vi "Eval X-Y-Z(a,t1,t2).vi"(5 "Variables":string[](array[string])=["t1", "t2"], 6 "Formulas":string[](array[string])=["", "", ""], 7 "Parameters":cluster{"name":string, "value":dbl}[](array[cluster]) {"value" format="%.2f"}, 8 "number of points":u32=25, 9 "End":dbl[](array[numeric])=[1.0, 1.0] format="%.2f", 10 "Start":dbl[](array[numeric])=[0.0, 0.0] format="%.2f") -> (0 "error":i32, 1 "ticks":u32, 2 "Z":dbl[](array[numeric]) format="%.2f", 3 "Y":dbl[](array[numeric]) format="%.2f", 4 "X":dbl[](array[numeric]) format="%.2f")   [LabVIEW 2020, in "NI_Gmath.lvlib"]
doc: "Describes a surface in 3D with two variables running over two different intervals."
uses:
  NI_Gmath.lvlib
panel:
  # "Example:\n\n number of points: 25 \n Start: 0.0 and 0.0\n End: 1.0 and 1.0\n Parameters: (a,1) and (b,2) \n Variables: t1 and t2\n Formulas: a*sin(t1) and a*cos(t1+t2) and b+exp(-t2)"
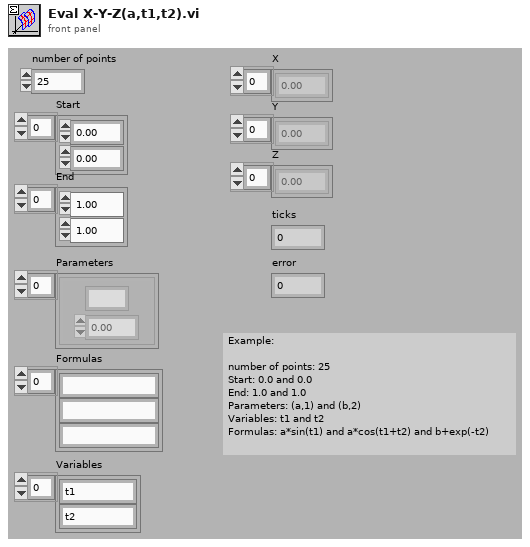
[diagram p1: front panel]
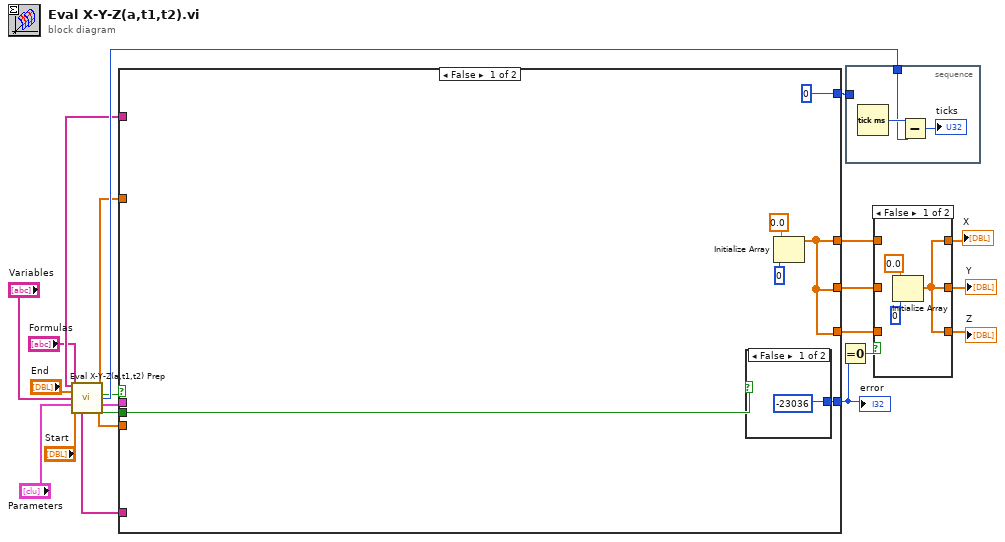
[diagram p0: block diagram]
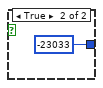
[diagram p3: hidden frame]
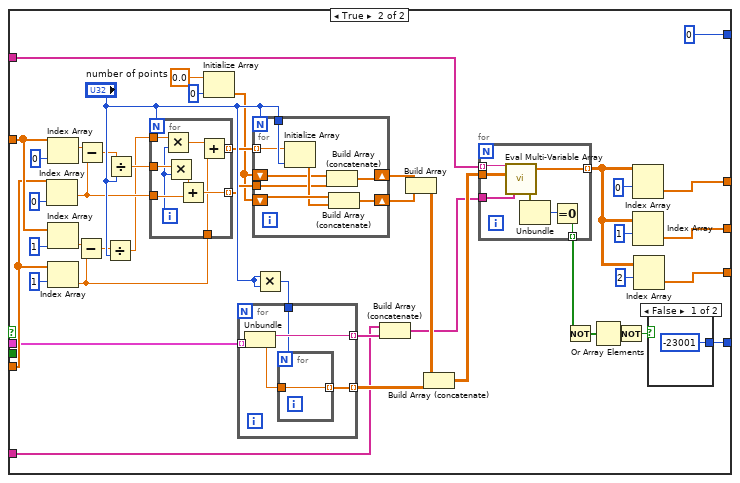
[diagram p4: hidden frame]
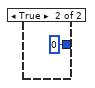
[diagram p5: hidden frame]
diagram:
  n1 = call "Eval X-Y-Z(a,t1,t2) Prep.vi"("End"="End", "Formulas"="Formulas", "Variables"="Variables", "Parameters"="Parameters", "Start"="Start") -> ("Formulas"=w17:string[], "End"=w19:dbl[], "time [msec]"=w21:u32, "error (general)"=w20:bool, "Variables"=w6:string[], "Start"=w18:dbl[], "Parameters"=w8:cluster{string, dbl}[], "specific error situation"=w7:bool)  [unwired: 3 in]
  n2 = case shown="False" w20 {
    tunnel: [0 0] -> w22
    tunnel: [w25 w43] -> w14
    tunnel: [w25 w42] -> w12
    tunnel: w19 -> [_ w41]
    tunnel: w18 -> [_ w40]
    tunnel: w6 -> [_ w39]
    tunnel: w8 -> [_ w38]
    tunnel: w17 -> [_ w37]
    tunnel: [w24 w34] -> w16
    tunnel: [w25 w33] -> w10
    tunnel: w7 -> [w23 _]
    frame False {
      n3 = case shown="False" w23 {
        tunnel: [-23036 -23033] -> w24
        frame False {
        }
        frame True {
        }
      }
      n4 = Initialize Array(0.0, 0) -> (w25:dbl[])
    }
    frame True {
      n5 = Index Array(array=w40, index=0) -> (element=w60:dbl)
      n6 = Index Array(array=w41, index=0) -> (element=w59:dbl)
      n7 = Index Array(array=w41, index=1) -> (element=w61:dbl)
      n8 = Index Array(array=w40, index=1) -> (element=w62:dbl)
      n9 = Subtract(x=w61, y=w62) -> (x-y=w51:dbl)
      n10 = Subtract(x=w59, y=w60) -> (x-y=w44:dbl)
      n11 = Divide(x=w51, y="number of points") -> (x/y=w53:dbl)
      n12 = Divide(x=w44, y="number of points") -> (x/y=w54:dbl)
      n13 = for {
        N: "number of points" -> [_]
        tunnel: w54 -> [w85]
        tunnel: w60 -> [w83]
        tunnel: [w82] -> w48 mode=indexing
        tunnel: w53 -> [w81]
        tunnel: w62 -> [w78]
        tunnel: [w77] -> w52 mode=indexing
        i -> [w80]
        n14 = Multiply(x=w81, y=w80) -> (x*y=w79:dbl)
        n15 = Multiply(x=w85, y=w80) -> (x*y=w84:dbl)
        n16 = Add(x=w84, y=w83) -> (x+y=w82:dbl)
        n17 = Add(x=w79, y=w78) -> (x+y=w77:dbl)
      }
      n18 = Initialize Array(0.0, 0) -> (w47:dbl[])
      n19 = for {
        N: "number of points" -> [_]
        tunnel: "number of points" -> [w93]
        tunnel: w52 -> [w92] mode=indexing
        shift-right: [w90] -> w50
        shift-left: w47 -> [w91]
        shift-right: [w88] -> w49
        shift-left: w47 -> [w87]
        tunnel: w48 -> [w86]
        n20 = Initialize Array(w92, w93) -> (w89:dbl[])
        n21 = Build Array (concatenate)(w87, w86) -> (w88:dbl[])
        n22 = Build Array (concatenate)(w91, w89) -> (w90:dbl[])
      }
      n23 = Multiply(x="number of points", y="number of points") -> (x*y=w71:u32)
      n24 = for {
        tunnel: [w105] -> w65 mode=indexing
        tunnel: [w103] -> w68 mode=indexing
        tunnel: w71 -> [w102]
        tunnel: w38 -> [w101] mode=indexing
        n25 = Unbundle(w101) -> (w105:string, w104:dbl)
        n26 = for {
          N: w102 -> [_]
          tunnel: [w106] -> w103 mode=indexing
          tunnel: w104 -> [w106]
        }
      }
      n27 = Build Array (concatenate)(w39, w65) -> (w66:string[])
      n28 = Build Array(w49, w50) -> (w67:dbl[][])
      n29 = Build Array (concatenate)(w67, w68) -> (w69:dbl[][])
      n30 = for {
        tunnel: w66 -> [w97]
        tunnel: w37 -> [w100] mode=indexing
        tunnel: w69 -> [w98]
        tunnel: [w99] -> w73 mode=indexing
        tunnel: [w94] -> w36 mode=indexing
        n31 = call "Eval Multi-Variable Array.vi"("Variables"=w97, "X Values"=w98, "formula"=w100) -> ("error out"=w96:errorcluster, "Y Values"=w99:dbl[])  [unwired: 1 in]
        n32 = Unbundle(w96) -> ("code"=w95:i32)  [unwired: 2 out]
        n33 = Equal To 0?(x=w95) -> (x = 0?=w94:bool)
      }
      n34 = Not(x=w36) -> (.not. x?=w32:bool[])
      n35 = Or Array Elements(Boolean array=w32) -> (logical OR=w35:bool)
      n36 = Not(x=w35) -> (.not. x?=w31:bool)
      n37 = Index Array(array=w73, index (row)=0) -> (element=w43:dbl[])  [unwired: 1 in]
      n38 = Index Array(array=w73, index (row)=1) -> (element=w42:dbl[])  [unwired: 1 in]
      n39 = Index Array(array=w73, index (row)=2) -> (element=w33:dbl[])  [unwired: 1 in]
      n40 = case shown="False" w31 {
        tunnel: [-23001 0] -> w34
        frame False {
        }
        frame True {
        }
      }
    }
  }
  "error" <- w16
  n41 = Equal To 0?(x=w16) -> (x = 0?=w15:bool)
  n42 = stacked-sequence {
    tunnel: w21 -> [w107]
    tunnel: w22 -> [_]
    frame #0 {
      n43 = Tick Count (ms)() -> (millisecond timer value=w109:u32)
      n44 = Subtract(x=w109, y=w107) -> (x-y=→"ticks":u32)
    }
  }
  n45 = case shown="False" w15 {
    tunnel: w14 -> [_ w115]
    tunnel: [w110 w115] -> w13
    tunnel: w12 -> [_ w114]
    tunnel: w10 -> [_ w113]
    tunnel: [w110 w113] -> w9
    tunnel: [w110 w114] -> w11
    frame False {
      n46 = Initialize Array(0.0, 0) -> (w110:dbl[])
    }
    frame True {
    }
  }
  "X" <- w13
  "Y" <- w11
  "Z" <- w9
